vi "Save CSV.vi"(5 "CSV FILE PATH Ref":refnum<vi>, 7 "MONITOR TABLE Ref":refnum<vi>, 8 "error in (no error)":errorcluster, 11 "Measurement UI Queue":refnum<queue>) -> (0 "error out":errorcluster)   [LabVIEW 2025, in "I2C Bus Monitor UI.lvlib"]
uses:
  I2C Bus Monitor UI.lvlib
  <vilib>/Utility/file.llb/Write Delimited Spreadsheet (string).vi
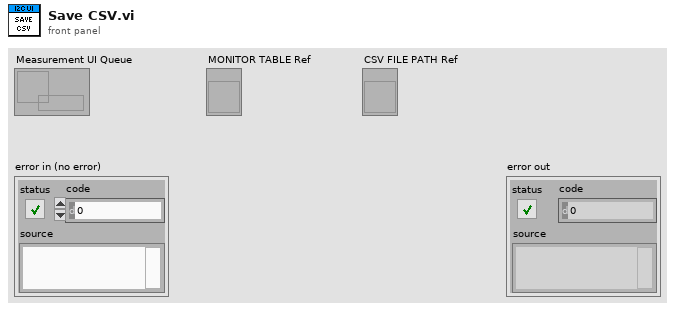
[diagram p1: front panel]
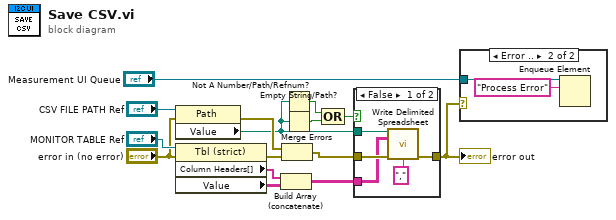
[diagram p0: block diagram]
diagram:
  n1 = property class="Path"(reference="CSV FILE PATH Ref", error in="error in (no error)") -> (error out=w15:errorcluster, "Value"=w4:path)  [unwired: 1 out]
  n2 = property class="Tbl (strict)"(reference="MONITOR TABLE Ref", error in="error in (no error)") -> (error out=w12:errorcluster, "Column Headers[]"=w8:string[], "Value"=w9:string[][])  [unwired: 1 out]
  n3 = Build Array (concatenate)(w8, w9) -> (w10:string[][])
  n4 = Merge Errors(w15, w12) -> (w11:errorcluster)
  n5 = Not A Number/Path/Refnum?(number/path/refnum=w4) -> (NaN/Path/Refnum?=w5:bool)
  n6 = Empty String/Path?(string/path=w4) -> (empty?=w7:bool)
  n7 = Compound Arithmetic op=OR(w5, w7) -> (w6:bool)
  n8 = case shown="False" w6 {
    tunnel: w4 -> [w20 _]
    tunnel: w11 -> [w19 w21]
    tunnel: [w17 w21] -> w2
    tunnel: w10 -> [w16 _]
    frame False {
      n9 = call-poly <vilib>:"Write Delimited Spreadsheet.vi"("file path (dialog if empty)"=w20, "2D data"=w16, "error in (no error)"=w19, "delimiter (\\t)"="," ("delimiter (\\t)")) -> ("error out"=w17:errorcluster)  [unwired: 10 in, 1 out]
    }
    frame True {
    }
  }
  "error out" <- w2
  n10 = case shown="Error .." w2 {
    tunnel: "Measurement UI Queue" -> [_ w23]
    frame No Error {
    }
    frame Error {
      n11 = Enqueue Element(queue=w23, element="Process Error") -> ()  [unwired: 2 in, 3 out]
    }
  }
